vi "RunningAverage-GetGroupData.vi"(8 "Error in":errorcluster, 9 "Enabled?":bool, 11 "Device Ref in":T1 format="%.0x") -> (0 "Error out":errorcluster, 2 "Group Data Array":T2(array[cluster]) {"VS Refs" format="%.0x"}, 3 "Device Ref out":T1=18446744073709551615 format="%.0x")   [LabVIEW 2017, in "Waveform-Processing-Custom-Device Shared.lvlib" / "Running Average.lvlib"]
uses:
  Running Average.lvlib
  <vilib>/NI Veristand/Custom Device API/Custom Device Item Ref.ctl
  Constants.vi
  <vilib>/NI Veristand/Custom Device API/Get Item Property (Dependent Node Pointer).vi
  System Explorer/Waveform-Processing-Custom-Device System Explorer.lvlib
  <vilib>/NI Veristand/Custom Device API/Custom Device API.lvlib
  Waveform-Processing-Custom-Device Shared.lvlib
  <vilib>/NI VeriStand/Custom Device Tools/Custom Device Utility Library/Custom Device Utility Library.lvlib
  <vilib>/NI Veristand/Custom Device Tools/Custom Device Utility Library/NI VeriStand - Search for Item by GUID.vi
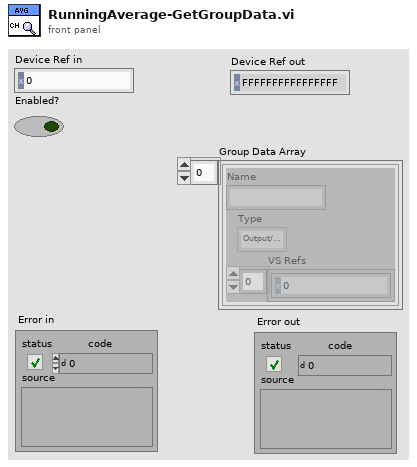
[diagram p1: front panel]
types:
  T1 = typedef "Custom Device API.lvlib/Custom Device Item Ref.ctl" = u64
  T2 = cluster{"Name":string, "Type":enum16{"Output/Write", "Input/Read", "Input/ReadWrite"}, "VS Refs":T1[]}[]
  T3 = enum16{"Output/Write", "Input/Read", "Input/ReadWrite"}
  T4 = cluster{"Name":string, "Type":enum16{"Output/Write", "Input/Read", "Input/ReadWrite"}, "VS Refs":T1[]}
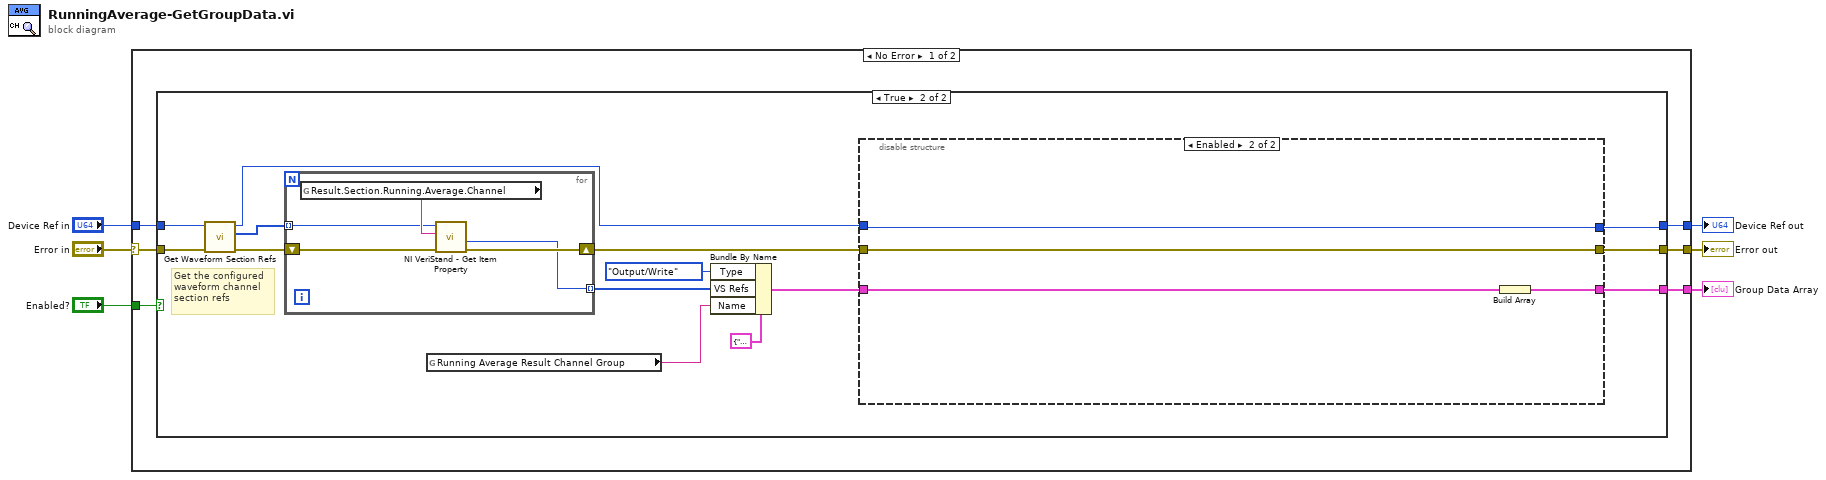
[diagram p0: block diagram]
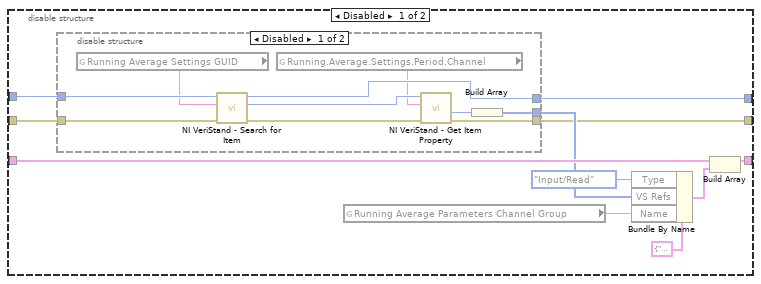
[diagram p3: hidden frame]
diagram:
  n1 = case shown="No Error" "Error in" {
    selector: "Error in" -> [w12 w62]
    tunnel: [w10 w62] -> w5
    tunnel: "Device Ref in" -> [w11 w61]
    tunnel: "Enabled?" -> [w9 _]
    tunnel: [w8 w61] -> w2
    tunnel: [w7 _] -> w1
    frame No Error {
      n2 = case shown="True" w9 {
        tunnel: w12 -> [w14 w28]
        tunnel: w11 -> [w13 w27]
        tunnel: [w14 w15] -> w10
        tunnel: [w13 w25] -> w8
        tunnel: [_ w18] -> w7
        frame False {
        }
        frame True {
          # "Get the configured\nwaveform channel\nsection refs"
          n3 = call "Get Waveform Section Refs.vi"("Error in"=w28, "Device Ref in"=w27) -> ("Error out"=w17:errorcluster, "Result Section Refs"=w26:T1[], "Device Ref out"=w23:T1)  [unwired: 7 in]
          n4 = for {
            tunnel: w26 -> [w56] mode=indexing
            shift-right: [w58] -> w16
            shift-left: w17 -> [w60]
            tunnel: [w57] -> w24 mode=indexing
            n5 = global read "Constants.vi" "Result.Section.Running.Average.Channel"() -> (w59:string)
            n6 = call-poly <vilib>:"NI VeriStand - Get Item Property.vi"("error in (no error)"=w60, "Property Name"=w59, "Item Ref in"=w56) -> ("error out"=w58:errorcluster, "Dependent Node Ref"=w57:T1)  [unwired: 5 in, 2 out]
          }
          n7 = global read "Constants.vi" "Running Average Result Channel Group"() -> (w22:string)
          n8 = Bundle By Name(cluster=T4 {"Name"="", "Type"=enum."Output/Write", "VS Refs"=[]} ("Group"), "Type"=T3."Output/Write", "VS Refs"=w24, "Name"=w22) -> (w19:T4)
          n9 = disable-structure shown="Enabled" {
            disable-tunnel: [w39 w53] -> w25
            disable-tunnel: w23 -> [w38 w53]
            disable-tunnel: w19 -> [w37 w55]
            disable-tunnel: [w36 w54] -> w18
            disable-tunnel: w16 -> [w30 w52]
            disable-tunnel: [w29 w52] -> w15
            frame Disabled {
              n10 = disable-structure shown="Disabled" {
                disable-tunnel: [w49 w51] -> w39
                disable-tunnel: w38 -> [w48 w51]
                disable-tunnel: [w44 _] -> w32
                disable-tunnel: w30 -> [w43 w50]
                disable-tunnel: [w41 w50] -> w29
                frame Disabled {
                  n11 = global read "Constants.vi" "Running Average Settings GUID"() -> (w47:string)
                  n12 = call-poly <vilib>:"NI VeriStand - Search for Item.vi"("error in"=w43, "Item GUID"=w47, "Section Ref in"=w48) -> ("error out"=w42:errorcluster, "Item Ref"=w46:T1, "Section Ref out"=w49:T1)  [unwired: 5 in, 1 out]
                  n13 = global read "Constants.vi" "Running.Average.Settings.Period.Channel"() -> (w40:string)
                  n14 = call-poly <vilib>:"NI VeriStand - Get Item Property.vi"("error in (no error)"=w42, "Property Name"=w40, "Item Ref in"=w46) -> ("error out"=w41:errorcluster, "Dependent Node Ref"=w45:T1)  [unwired: 5 in, 2 out]
                  n15 = Build Array(w45) -> (w44:T1[])
                }
                frame Enabled {
                }
              }
              n16 = global read "Constants.vi" "Running Average Parameters Channel Group"() -> (w33:string)
              n17 = Bundle By Name(cluster=T4 {"Name"="", "Type"=enum."Output/Write", "VS Refs"=[]} ("Group"), "Type"=T3."Input/Read", "VS Refs"=w32, "Name"=w33) -> (w31:T4)
              n18 = Build Array(w37, w31) -> (w36:T2)
            }
            frame Enabled {
              n19 = Build Array(w55) -> (w54:T2)
            }
          }
        }
      }
    }
    frame Error {
    }
  }
  "Error out" <- w5
  "Device Ref out" <- w2
  "Group Data Array" <- w1
